vi "FA_StringToSpecialType.vi"(0 "Special Type String":string) -> (6 "Special Type Enum":T1)   [LabVIEW 2014]
uses:
  FA_LSSpecialTypes.ctl
  FA_LocalStore.lvlib
panel:
  out "Error Out":errorcluster
  in  "Error In":errorcluster
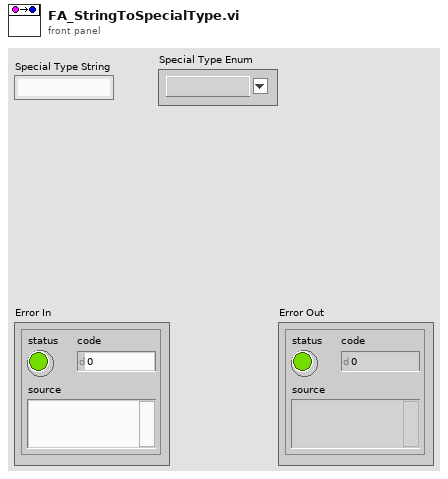
[diagram p1: front panel]
types:
  T1 = typedef "FA_LocalStore.lvlib/FA_LSSpecialTypes.ctl" = string
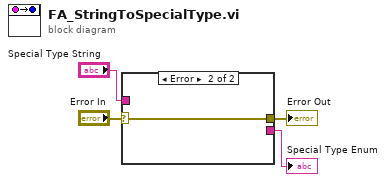
[diagram p0: block diagram]
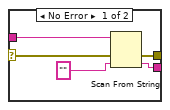
[diagram p2: hidden frame]
diagram:
  n1 = case shown="Error" "Error In" {
    selector: "Error In" -> [w6 w10]
    tunnel: [w5 w10] -> w1
    tunnel: "Special Type String" -> [w8 _]
    tunnel: [w7 _] -> w3
    frame No Error {
      n2 = Scan From String(input string=w8, error in=w6, default 1=T1 "" ("Special Type")) -> (error out=w5:errorcluster, output 1=w7:T1)  [unwired: 2 in, 2 out]
    }
    frame Error {
    }
  }
  "Special Type Enum" <- w3
  "Error Out" <- w1
